vi "Write to Property Bag.vi"(8 "error in (no error)":errorcluster, 9 "Prototype in":variant, 10 "Node":string, 11 "INI Deserializer in":refnum<class "INI Deserializer.lvclass">) -> (0 "error out":errorcluster, 1 "Data out":variant, 3 "INI Deserializer out":refnum<class "INI Deserializer.lvclass">)   [LabVIEW 2014, in "INI Deserializer.lvclass"]
uses:
  INI Deserializer.lvclass
  INI Deserializer.lvclass/INI Deserializer.ctl
  <vilib>/Utility/error.llb/Error Cluster From Error Code.vi
  <vilib>/Utility/config.llb/Read Key (Boolean).vi
  <vilib>/Utility/config.llb/Read Key (Double).vi
  <vilib>/Utility/config.llb/Read Key (I32).vi
  <vilib>/Utility/config.llb/Read Key (Path).vi
  <vilib>/Utility/config.llb/Read Key (String).vi
  <vilib>/Utility/config.llb/Read Key (U32).vi
  <vilib>/ErrorRing/Error Ring.xnode
  <vilib>/Utility/VariantDataType/VariantType.lvlib
  <vilib>/Utility/config.llb/NI_LVConfig.lvlib
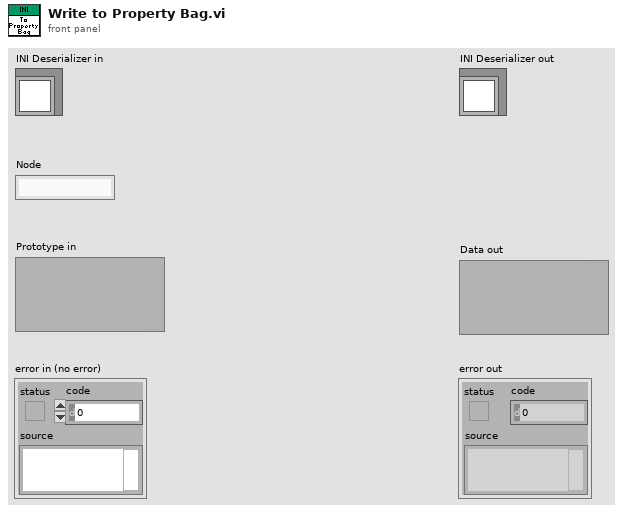
[diagram p1: front panel]
types:
  T1 = typedef "NI_LVConfig.lvlib/Config Data RefNum.ctl" = refnum<k1>
  T2 = typedef "VariantType.lvlib/Type.ctl" = enum8{"Invalid Type", "Void", "I8", "I16", "I32", "I64", "U8", "U16", "U32", "U64", "Single Float", "Double Float", "Extended Float", "Single Complex", "Double Complex", "Extended Complex", "Enum U8", "Enum U16", "Enum U32", "Enum U64", "Single Float With Unit", "Double Float With Unit", "Extended Float With Unit", "Single Complex with Unit", "Double Complex with Unit", "Extended Complex with Unit", "Boolean", "String", "Path", "Picture", "Tag", "Array", "Cluster", "Variant", "LV Variant", "Waveform", "Timestamp", "Digital Waveform", "Digital Data", "ExpressData", "Refnum", "External Data", "VI", "Poly VI", "LabVIEW Class Instance", "Fixed Point"}
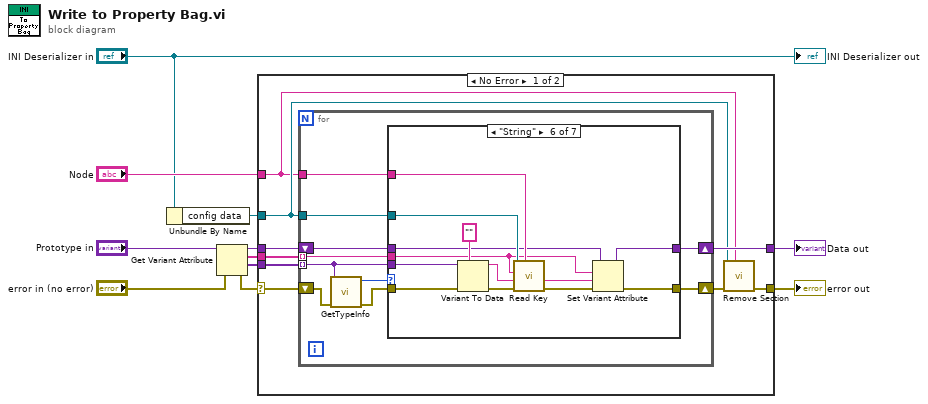
[diagram p0: block diagram]
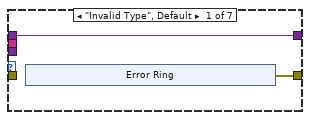
[diagram p2: hidden frame]
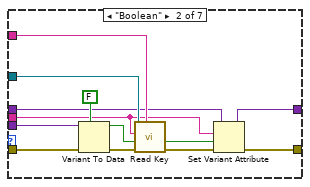
[diagram p3: hidden frame]
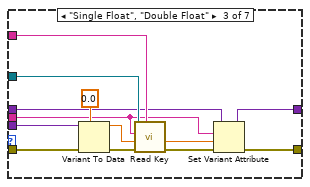
[diagram p4: hidden frame]
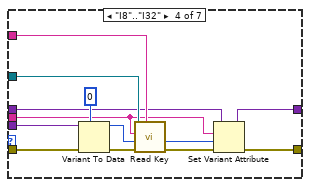
[diagram p5: hidden frame]
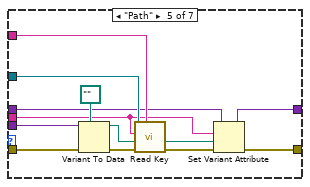
[diagram p6: hidden frame]
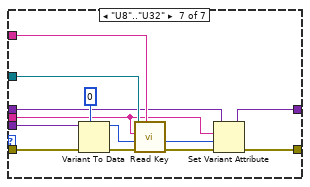
[diagram p7: hidden frame]
diagram:
  n1 = Unbundle By Name("INI Deserializer in") -> ("config data"=w10:T1)
  n2 = Get Variant Attribute(Variant="Prototype in", error in="error in (no error)") -> (duplicate Variant=w5:variant, names=w9:string[], values=w11:variant[], error out=w1:errorcluster)  [unwired: 2 in]
  n3 = case shown="No Error" w1 {
    selector: w1 -> [w17 w116]
    tunnel: w11 -> [w20 _]
    tunnel: w10 -> [w13 _]
    tunnel: "Node" -> [w12 _]
    tunnel: w9 -> [w19 _]
    tunnel: [w14 w116] -> w7
    tunnel: w5 -> [w16 w115]
    tunnel: [w15 w115] -> w4
    frame No Error {
      n4 = for {
        tunnel: w20 -> [w21] mode=indexing
        tunnel: w13 -> [w29]
        tunnel: w12 -> [w28]
        tunnel: w19 -> [w27] mode=indexing
        shift-right: [w25] -> w18
        shift-left: w17 -> [w22]
        shift-right: [w23] -> w15
        shift-left: w16 -> [w24]
        n5 = call <vilib>:"GetTypeInfo.vi"("error in (no error)"=w22, "Variant"=w21) -> ("error out"=w26:errorcluster, "Type Enum"=w30:T2)  [unwired: 5 in, 3 out]
        n6 = case shown="\"String\"" w30 {
          tunnel: w21 -> [_ w48 w62 w74 w88 w101 w113]
          tunnel: w29 -> [_ w46 w60 w72 w86 w99 w111]
          tunnel: w28 -> [_ w45 w59 w71 w85 w98 w110]
          tunnel: w27 -> [_ w40 w51 w64 w76 w89 w102]
          tunnel: w26 -> [_ w43 w57 w70 w83 w96 w108]
          tunnel: [w32 w41 w54 w67 w80 w93 w106] -> w25
          tunnel: [w31 w38 w52 w65 w78 w91 w104] -> w23
          tunnel: w24 -> [w31 w39 w53 w66 w79 w92 w105]
          frame "Invalid Type", Default {
            n7 = xnode "Error Ring"() -> ("error out"=w32:errorcluster)
          }
          frame "Boolean" {
            n8 = Variant To Data(error in=w43, type=FALSE, Variant=w48) -> (data=w49:bool, error out=w47:errorcluster)
            n9 = call-poly <vilib>:"Read Key.vi"("section"=w45, "error in (no error)"=w47, "default value"=w49, "key"=w40, "refnum"=w46) -> ("error out"=w42:errorcluster, "value"=w37:bool)  [unwired: 3 in, 2 out]
            n10 = Set Variant Attribute(Variant=w39, name=w40, value=w37, error in=w42) -> (Variant out=w38:variant, error out=w41:errorcluster)  [unwired: 1 out]
          }
          frame "Single Float", "Double Float" {
            n11 = Variant To Data(error in=w57, type=0.0, Variant=w62) -> (data=w55:dbl, error out=w61:errorcluster)
            n12 = call-poly <vilib>:"Read Key.vi"("section"=w59, "error in (no error)"=w61, "default value"=w55, "key"=w51, "refnum"=w60) -> ("error out"=w56:errorcluster, "value"=w50:dbl)  [unwired: 3 in, 2 out]
            n13 = Set Variant Attribute(Variant=w53, name=w51, value=w50, error in=w56) -> (Variant out=w52:variant, error out=w54:errorcluster)  [unwired: 1 out]
          }
          frame "I8".."I32" {
            n14 = Variant To Data(error in=w70, type=0 ("value"), Variant=w74) -> (data=w68:i32, error out=w73:errorcluster)
            n15 = call-poly <vilib>:"Read Key.vi"("section"=w71, "error in (no error)"=w73, "default value"=w68, "key"=w64, "refnum"=w72) -> ("error out"=w69:errorcluster, "value"=w63:i32)  [unwired: 3 in, 2 out]
            n16 = Set Variant Attribute(Variant=w66, name=w64, value=w63, error in=w69) -> (Variant out=w65:variant, error out=w67:errorcluster)  [unwired: 1 out]
          }
          frame "Path" {
            n17 = Variant To Data(error in=w83, type=path "", Variant=w88) -> (data=w81:path, error out=w87:errorcluster)
            n18 = call-poly <vilib>:"Read Key.vi"("section"=w85, "error in (no error)"=w87, "default value"=w81, "key"=w76, "refnum"=w86) -> ("error out"=w82:errorcluster, "value"=w77:path)  [unwired: 3 in, 2 out]
            n19 = Set Variant Attribute(Variant=w79, name=w76, value=w77, error in=w82) -> (Variant out=w78:variant, error out=w80:errorcluster)  [unwired: 1 out]
          }
          frame "String" {
            n20 = Variant To Data(error in=w96, type="", Variant=w101) -> (data=w94:string, error out=w100:errorcluster)
            n21 = call-poly <vilib>:"Read Key.vi"("section"=w98, "error in (no error)"=w100, "default value"=w94, "key"=w89, "refnum"=w99) -> ("error out"=w95:errorcluster, "value"=w90:string)  [unwired: 3 in, 2 out]
            n22 = Set Variant Attribute(Variant=w92, name=w89, value=w90, error in=w95) -> (Variant out=w91:variant, error out=w93:errorcluster)  [unwired: 1 out]
          }
          frame "U8".."U32" {
            n23 = Variant To Data(error in=w108, type=u32 0 ("value"), Variant=w113) -> (data=w107:u32, error out=w112:errorcluster)
            n24 = call-poly <vilib>:"Read Key.vi"("section"=w110, "error in (no error)"=w112, "default value"=w107, "key"=w102, "refnum"=w111) -> ("error out"=w109:errorcluster, "value"=w103:u32)  [unwired: 3 in, 2 out]
            n25 = Set Variant Attribute(Variant=w105, name=w102, value=w103, error in=w109) -> (Variant out=w104:variant, error out=w106:errorcluster)  [unwired: 1 out]
          }
        }
      }
      n26 = call <vilib>:"Remove Section.vi"("section"=w12, "error in (no error)"=w18, "refnum"=w13) -> ("error out"=w14:errorcluster)  [unwired: 6 in, 2 out]
    }
    frame Error {
    }
  }
  "error out" <- w7
  "Data out" <- w4
  "INI Deserializer out" <- "INI Deserializer in"
